vi "LogTextBuffer.vi"(8 "buffer lines":i32=100, 10 "new message":string) -> (2 "log":string)   [LabVIEW 2014]
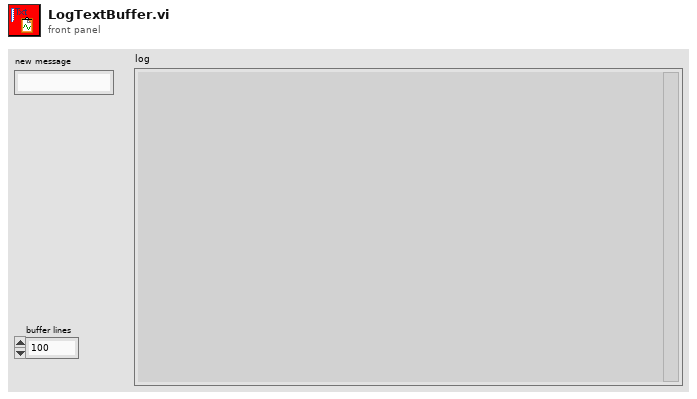
[diagram p1: front panel]
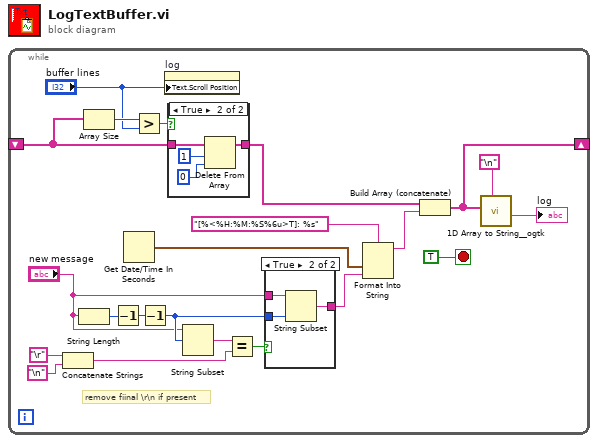
[diagram p0: block diagram]
diagram:
  n1 = while {
    shift-right: [w20] -> _
    shift-left: _ -> [w15]
    stop <- TRUE stop-if-true
    # "remove fiinal \\r\\n if present"
    n2 = Concatenate Strings("\r", "\n") -> (w5:string)
    n3 = String Length(string="new message") -> (length=w6:i32)
    n4 = Array Size(array=w15) -> (size(s)=w18:i32)
    n5 = Decrement(x=w6) -> (x-1=w7:i32)
    n6 = Get Date/Time In Seconds() -> (seconds since 1Jan1904=w12:timestamp)
    n7 = Greater?(x=w18, y="buffer lines") -> (0:w16:bool)
    n8 = Decrement(x=w7) -> (x-1=w2:i32)
    n9 = property on="log" class="Str"("Text.Scroll Position"="buffer lines") -> ()  [unwired: 2 in, 2 out]
    n10 = case shown="True" w16 {
      tunnel: w15 -> [w27 w31]
      tunnel: [w27 w30] -> w14
      frame False {
      }
      frame True {
        n11 = Delete From Array(array=w31, length=1, index=0) -> (array with subset deleted=w30:string[])  [unwired: 1 out]
      }
    }
    n12 = String Subset(string="new message", offset (0)=w2) -> (substring=w8:string)  [unwired: 1 in]
    n13 = Equal?(x=w8, y=w5) -> (x = y?=w4:bool)
    n14 = case shown="True" w4 {
      tunnel: "new message" -> [w23 w26]
      tunnel: [w23 w25] -> w3
      tunnel: w2 -> [_ w24]
      frame False {
      }
      frame True {
        n15 = String Subset(string=w26, length (rest)=w24) -> (substring=w25:string)  [unwired: 1 in]
      }
    }
    n16 = Format Into String(format string="[%<%H:%M:%S%6u>T]: %s", w12, w3) -> (resulting string=w13:string)  [unwired: 2 in, 1 out]
    n17 = Build Array (concatenate)(w14, w13) -> (w20:string[])
    n18 = call "1D Array to String__ogtk.vi"("delimiter (Tab)"="\n", "Array of Strings"=w20) -> ("delimited string"=→"log":string)  [unwired: 9 in]
  }
